vi "纳清叶绿素a电极校准.vi"() -> ()   [LabVIEW 2016, in "斯坦道多参数.lvlib"]
uses:
  <vilib>/Utility/miscctls.llb/LVPointTypeDef.ctl
  <vilib>/Utility/miscctls.llb/LVPositionTypeDef.ctl
  <vilib>/Analysis/NI_AALBase.lvlib
panel:
  out "滤波设定":sgl
  in  "量程":u16(ring) items=["0-500", "0-50"]
  out "第三点信号值":dbl
  out "第二点信号值":dbl
  out "第一点信号值":dbl
  out "报警信息":string
  out "通讯状态":string
  out "第三点校准值":dbl
  out "标液3":sgl
  out "第二点校准值":dbl
  out "第一点校准值":dbl
  in  "校准停止":bool
  in  "校准启动":bool
  in  "校准模式":u16(ring)=1 items=["两点校准", "单点校准", "三点校准"]
  out "最小值":sgl format="%#.2f"
  out "最大值":sgl format="%#.2f"
  out "波形图表":dbl(graph) caption="历史曲线"
  out "mean":dbl caption="均值" format="%#.2f"
  out "standard deviation":dbl caption="标准差" format="%#.2f"
  out "变异系数":dbl format="%#.6f"
  out "测量值":sgl format="%#.2f"
  out "提示":string
  out "标液2":sgl
  out "标液1":sgl
  out "原始光强数值":u16 caption="信号值"
  out "温度":dbl format="%#.2f"
  # "叶绿素a电极设定"
  # "℃"
  # "μg/L"
  # "μg/L"
  # "请选择校准模式:"
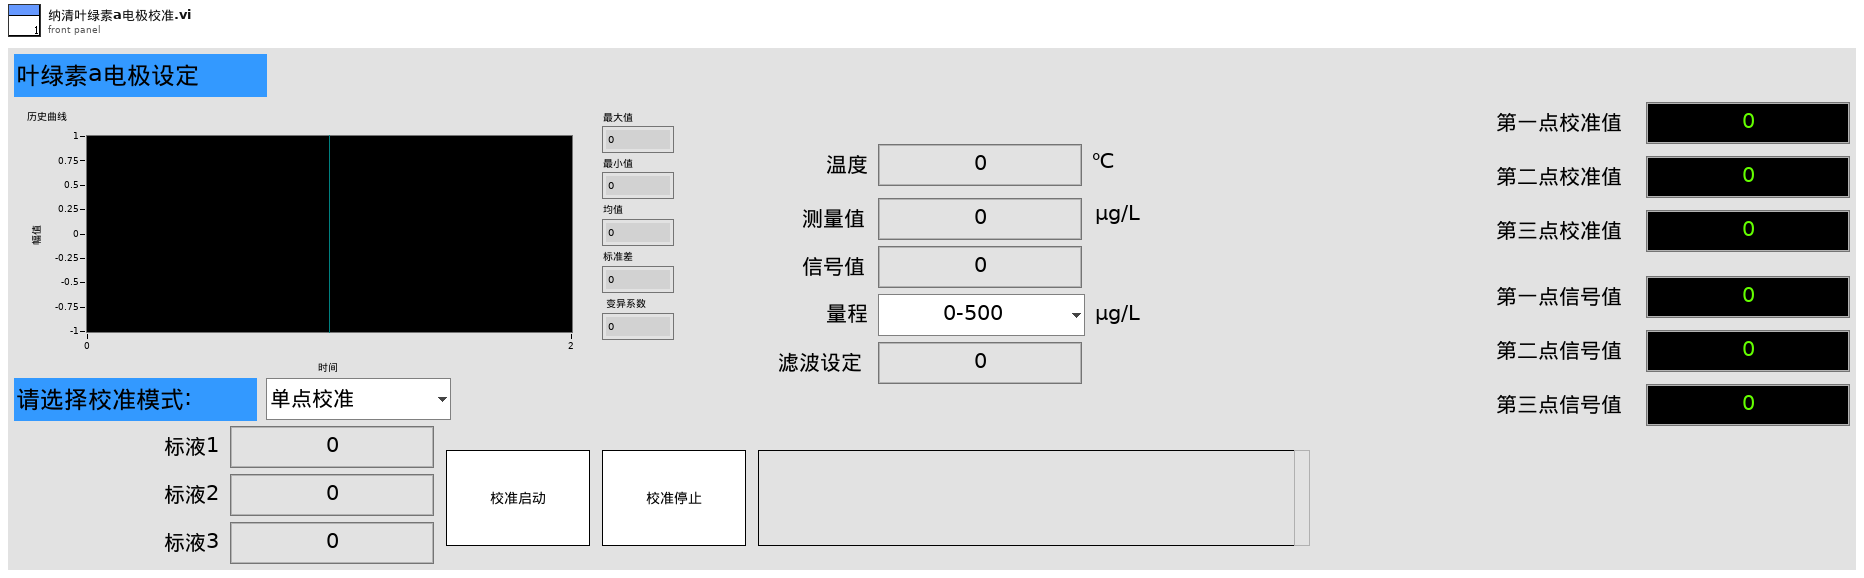
[diagram p1: front panel]
types:
  T1 = enum16{"pH", "DO", "Cond", "Turb", "ORP", "叶绿素a", "藻密度"}
  T2 = typedef "LVPointTypeDef.ctl" = cluster{"Horizontal":i16, "Vertical":i16}
  T3 = cluster{"报警码":u16, "叶绿素a":sgl, "温度数据":sgl, "原始光强数值":u16, "量程":u16, "平均次数":u16, "清扫模式":u16, "清扫次数":u16, "清扫间隔分钟":u16, "0X000B_NC":string, "产品名称":string, "序列号":string, "硬件版本":string, "软件版本":string, "通讯地址":u16, "波特率":u16, "设备类型":u16, "0X0026_NC":string, "校准量程":u16, "第一点原始光强":u16, "第一点校准数据":sgl, "第二点原始光强":u16, "第二点校准数据":sgl, "第三点原始光强":u16, "第三点校准数据":sgl, "探头校准命令":u16, "温度校准参数":sgl, "温度校准命令":u16}
  T4 = cluster{"pH":u32, "DO":u32, "Cond":u32, "Turb":u32, "叶绿素a":u32, "藻密度":u32, "ORP":u32}
  T5 = typedef "LVPositionTypeDef.ctl" = cluster{"Left":i32, "Top":i32}
  T6 = enum8{"Enabled", "Disabled", "Disabled and Grayed Out"}
  T7 = cluster{"ph":bool, "DO":bool, "Cond":bool, "Turb":bool, "叶绿素a":bool, "藻密度":bool, "ORP":bool}
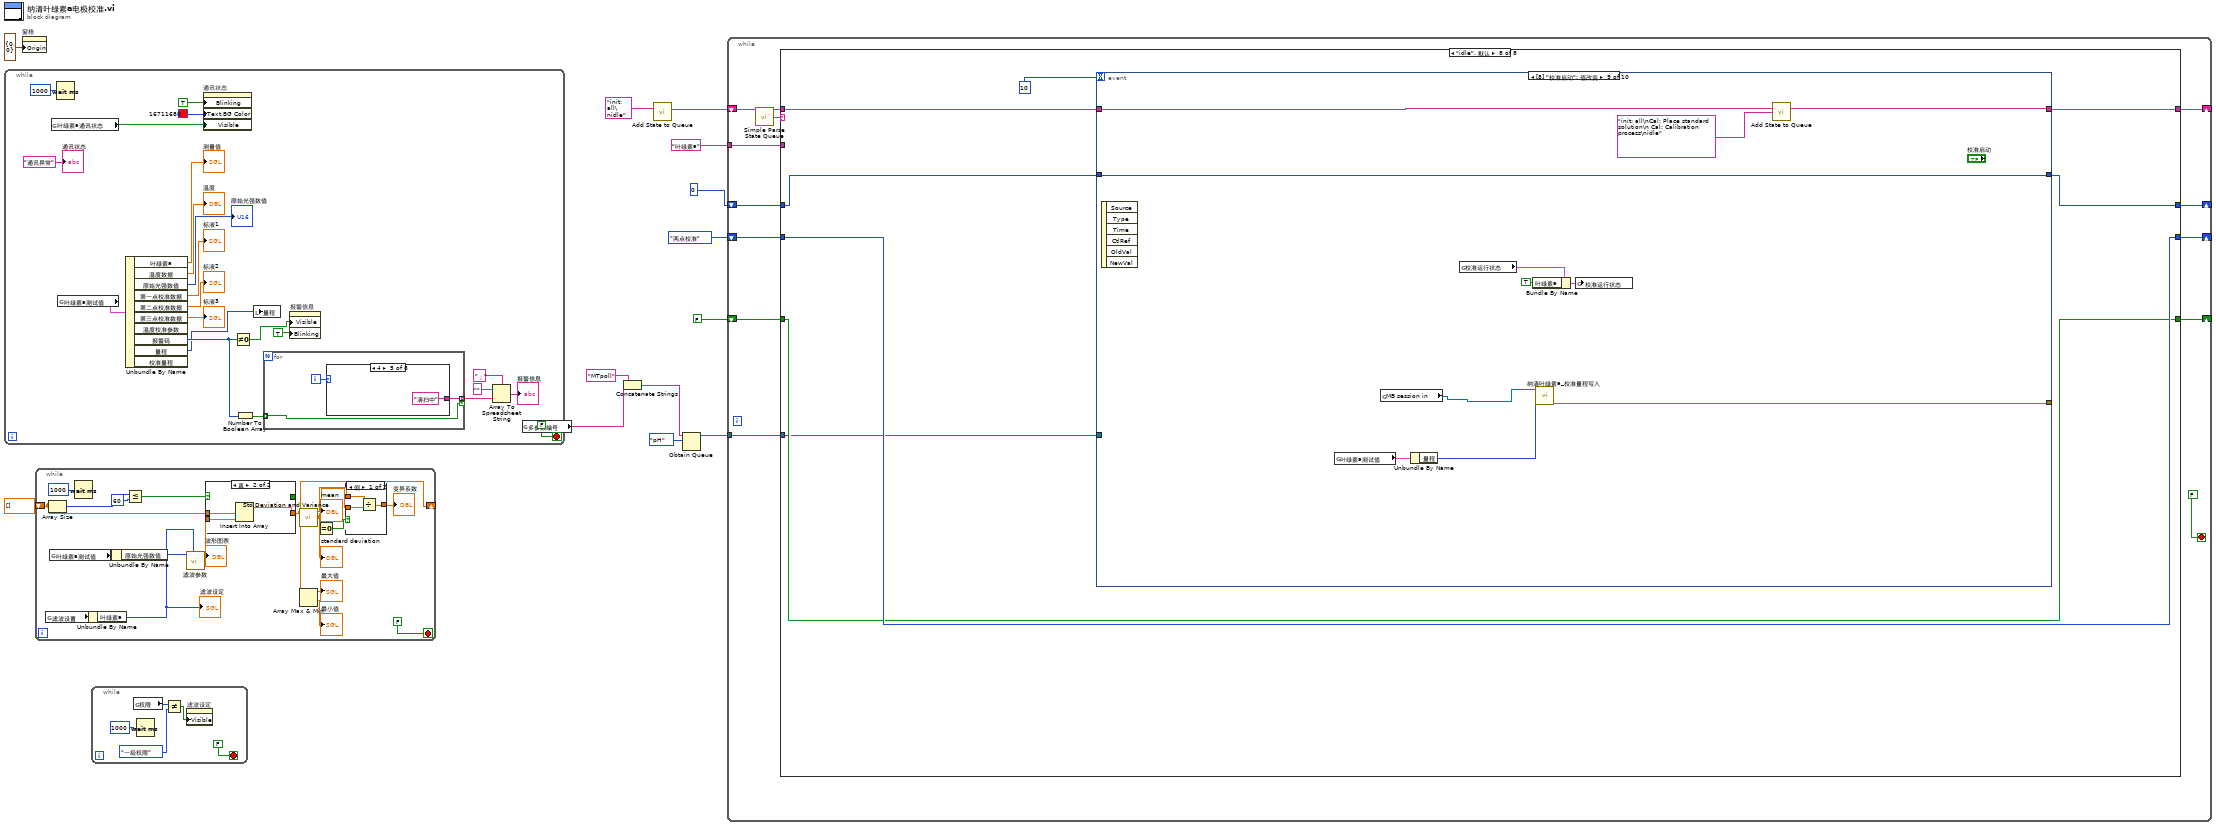
[diagram p0: block diagram]
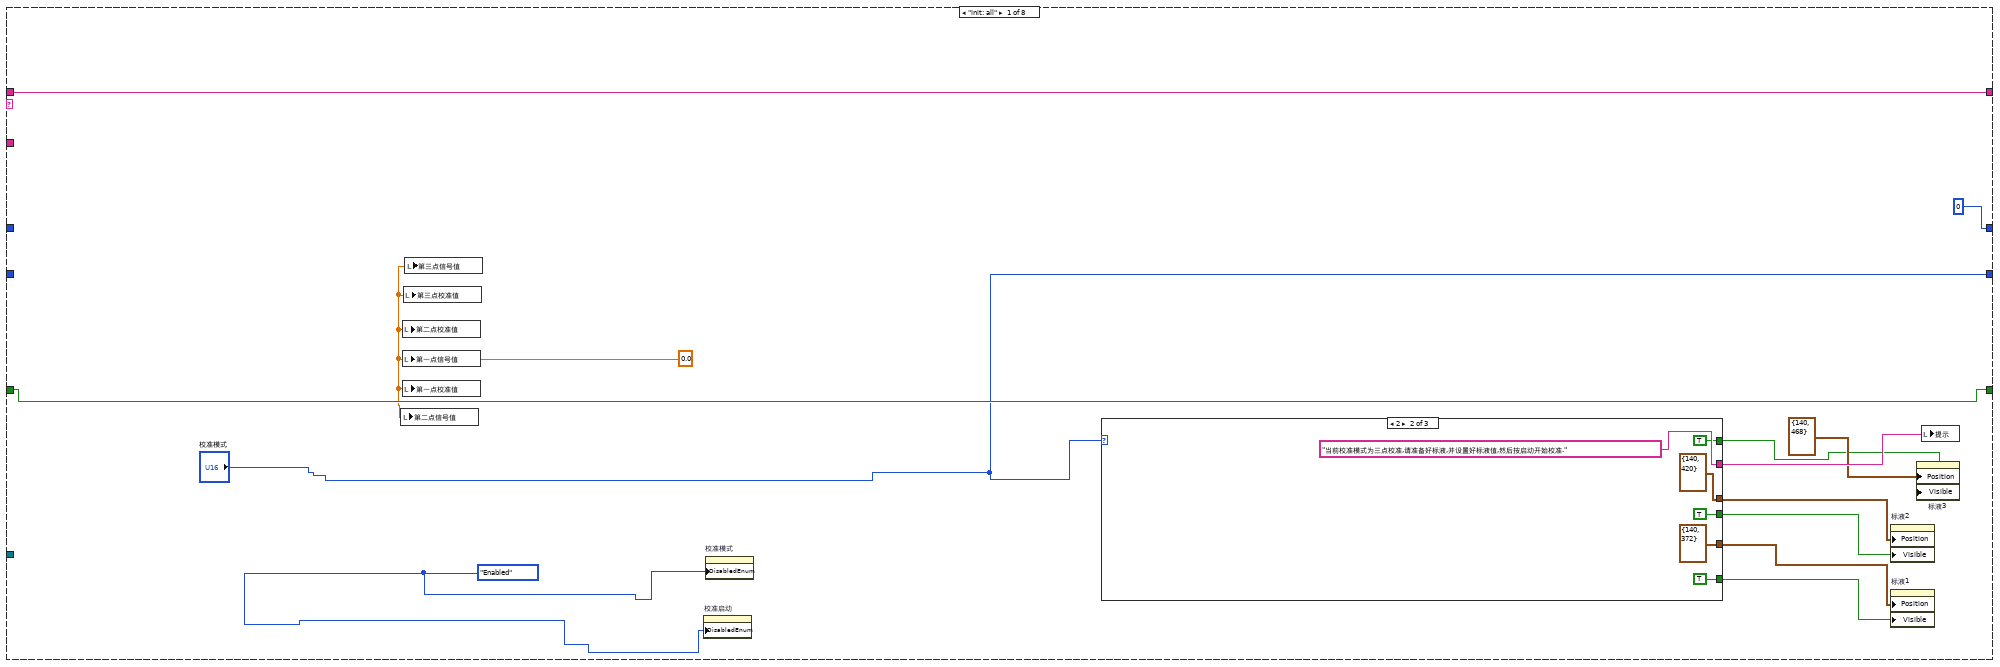
[diagram p2: hidden frame]
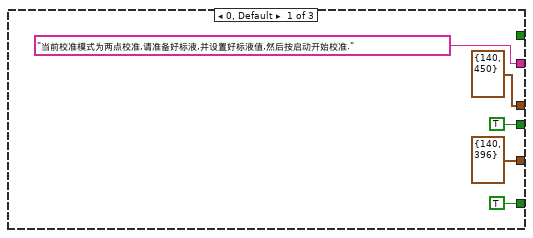
[diagram p3: hidden frame]
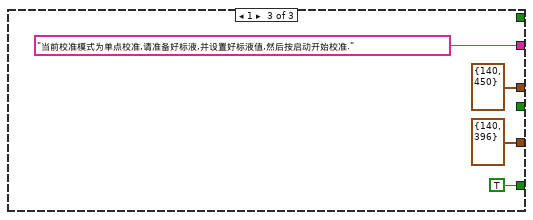
[diagram p4: hidden frame]
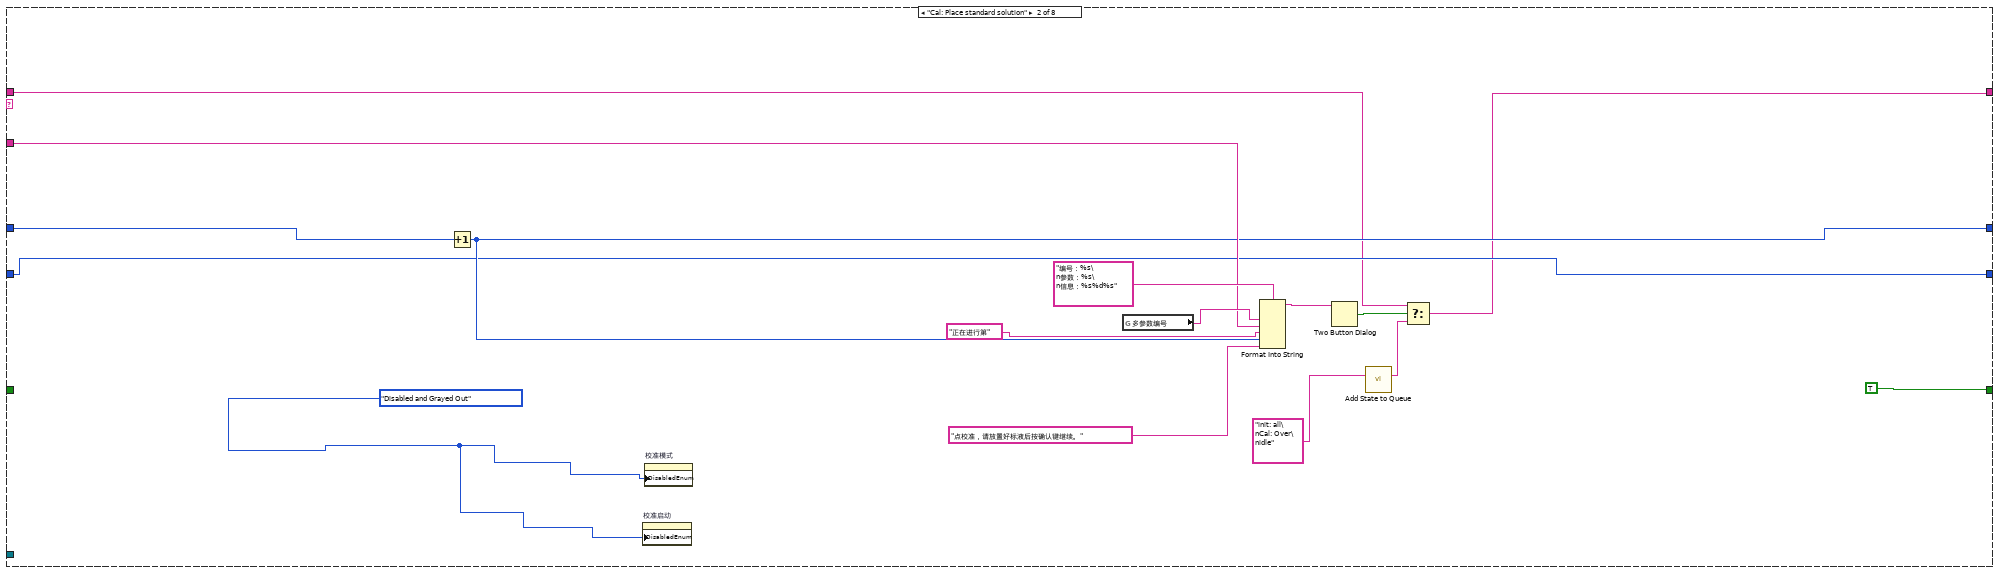
[diagram p5: hidden frame]
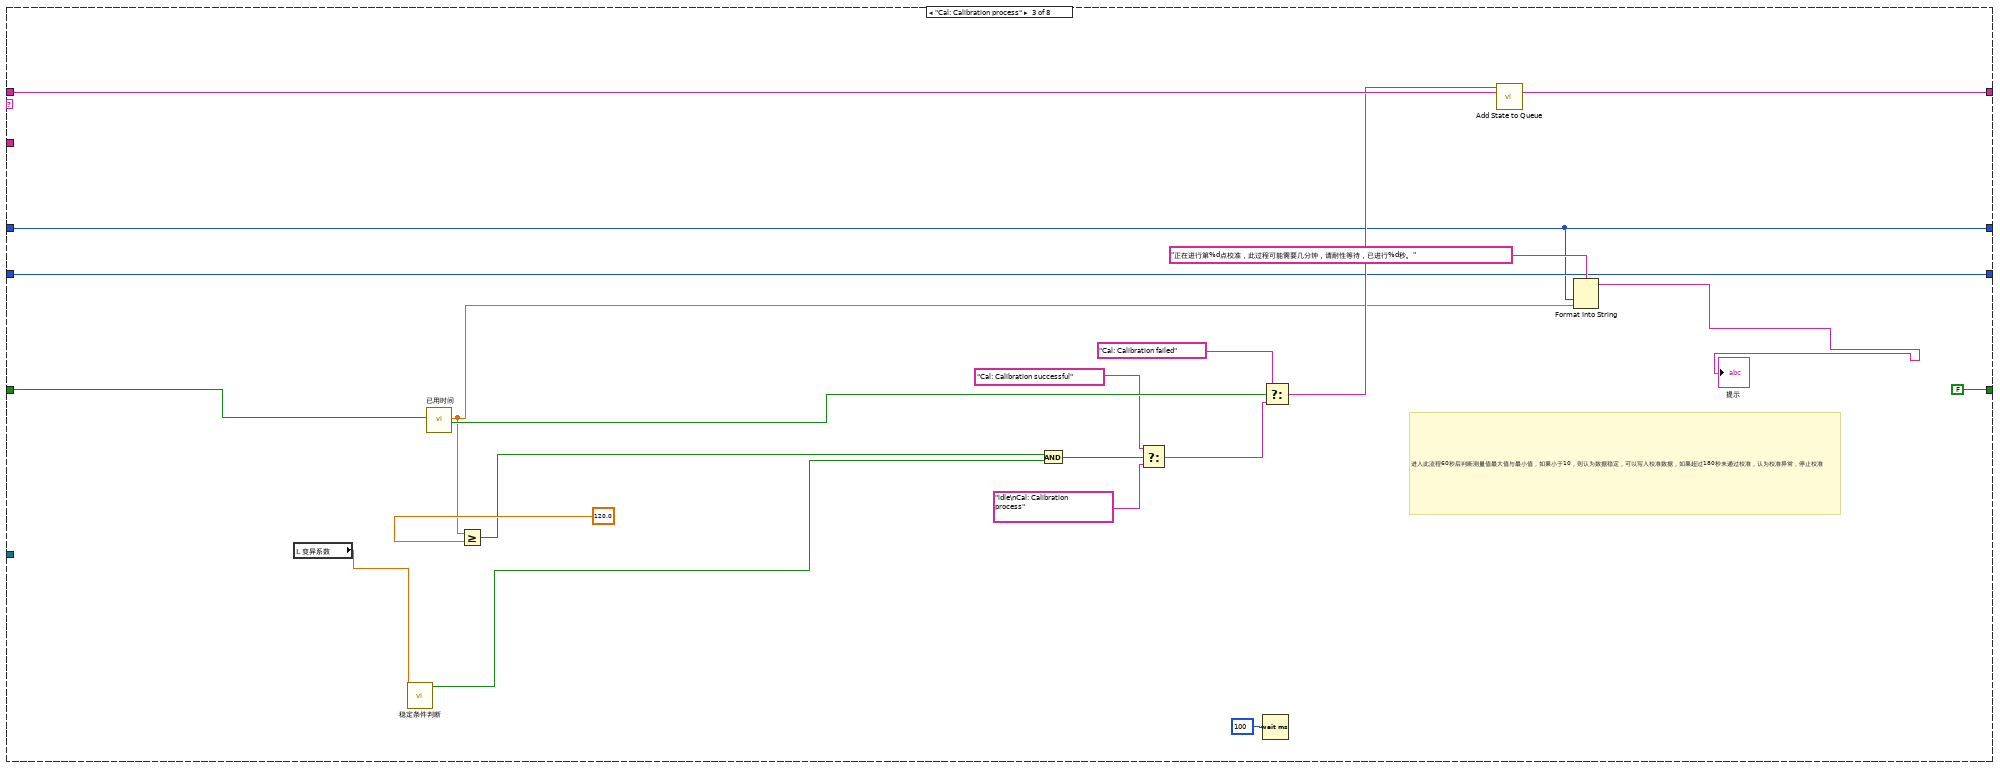
[diagram p6: hidden frame]
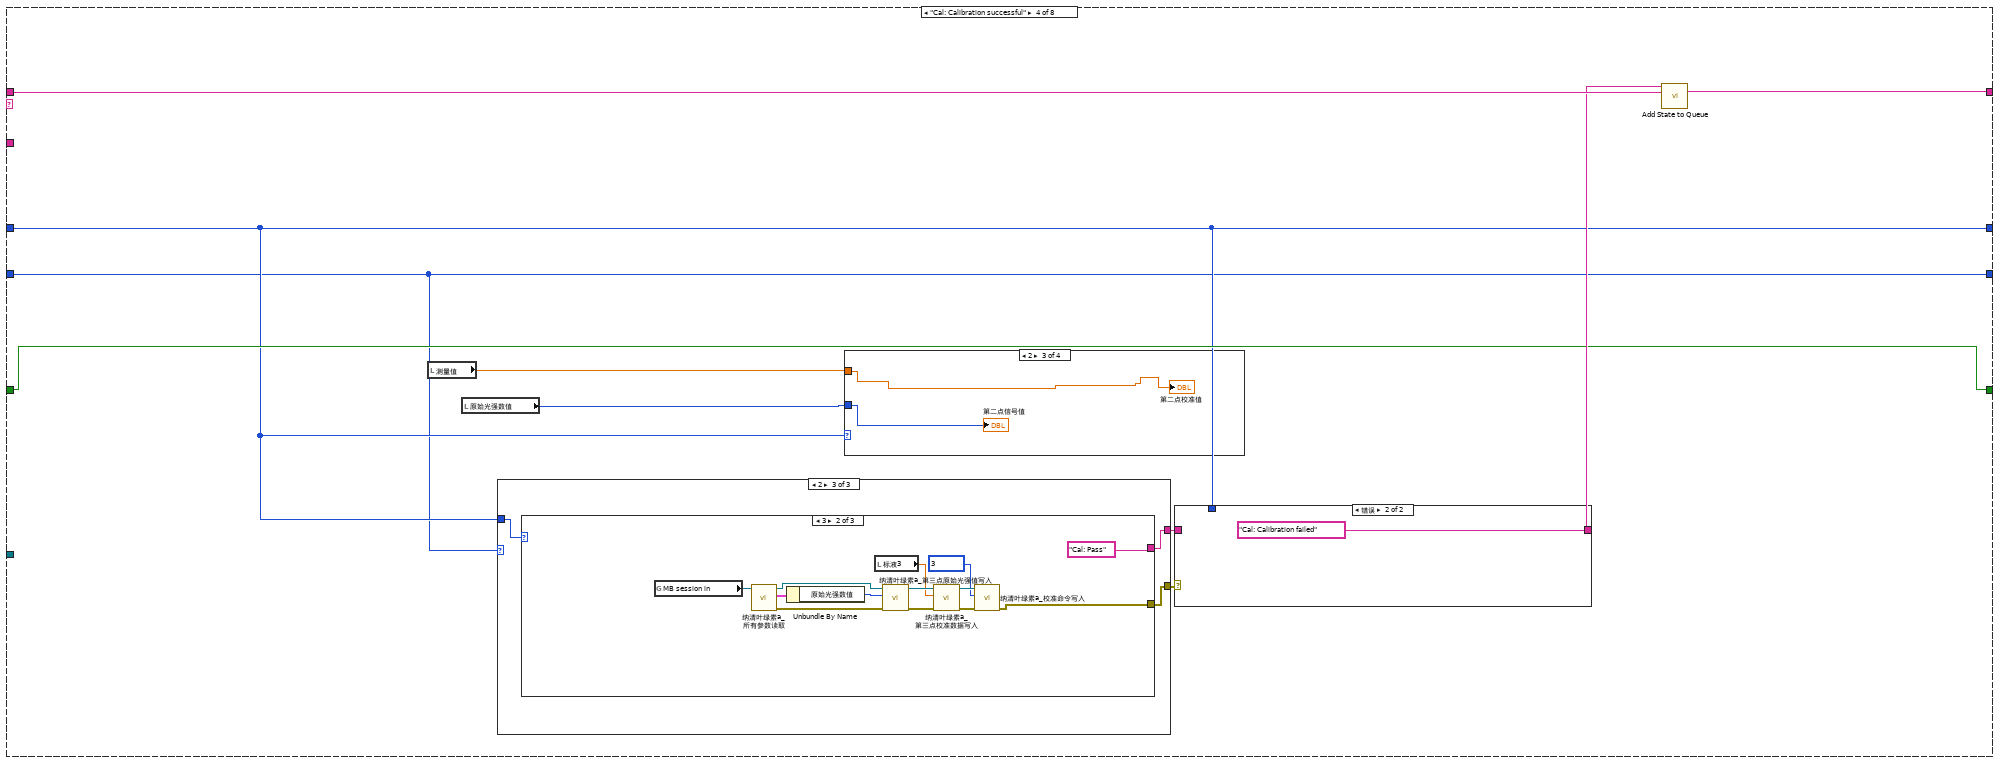
[diagram p7: hidden frame]
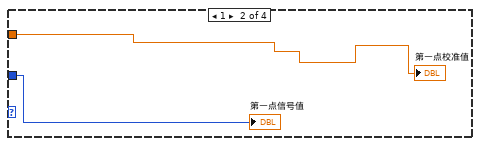
[diagram p9: hidden frame]
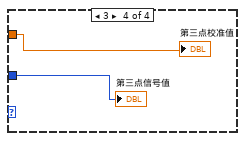
[diagram p10: hidden frame]
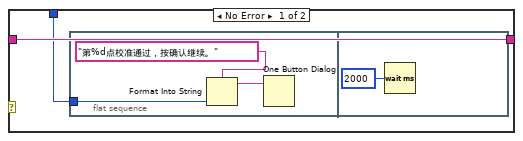
[diagram p11: hidden frame]
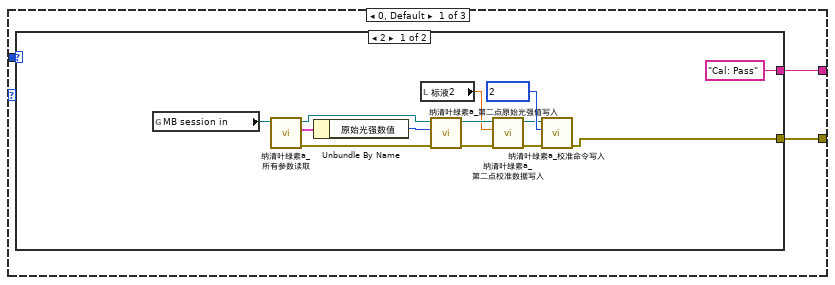
[diagram p12: hidden frame]
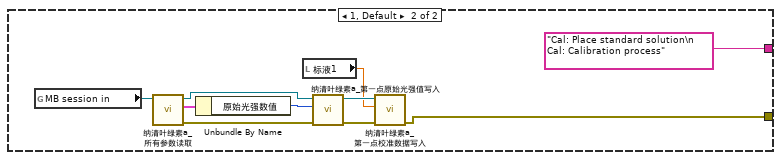
[diagram p13: hidden frame]
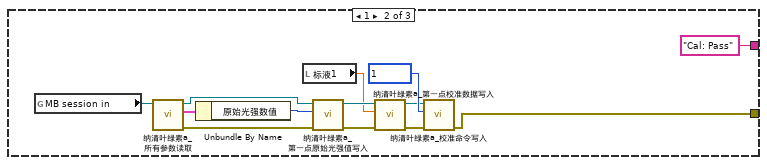
[diagram p14: hidden frame]
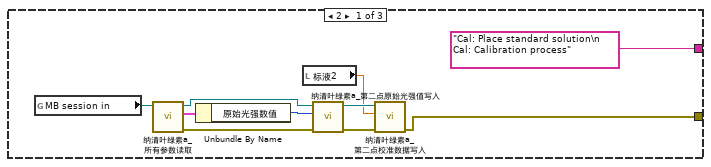
[diagram p15: hidden frame]
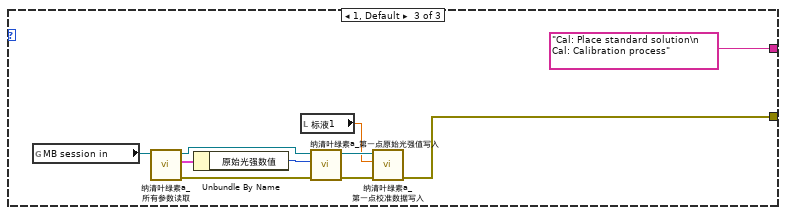
[diagram p16: hidden frame]
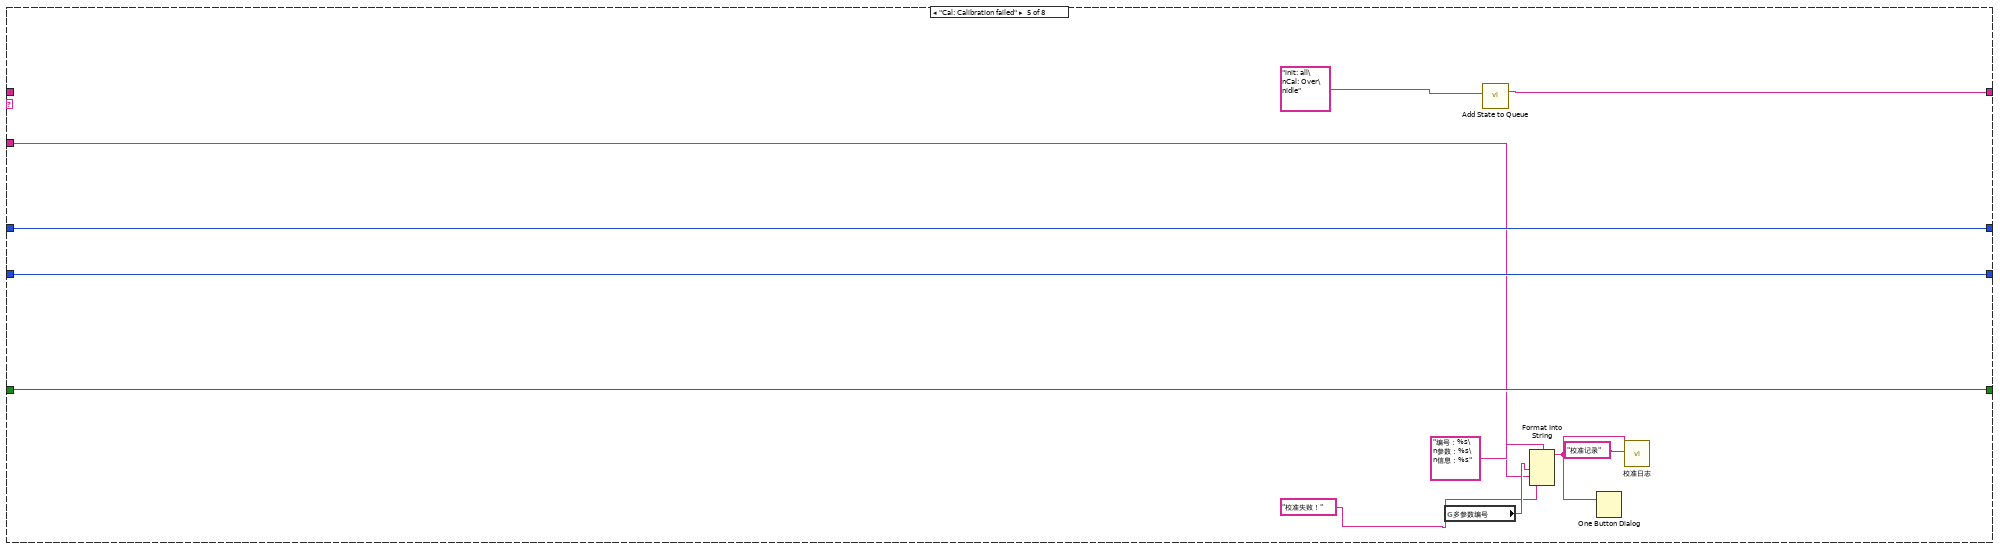
[diagram p17: hidden frame]
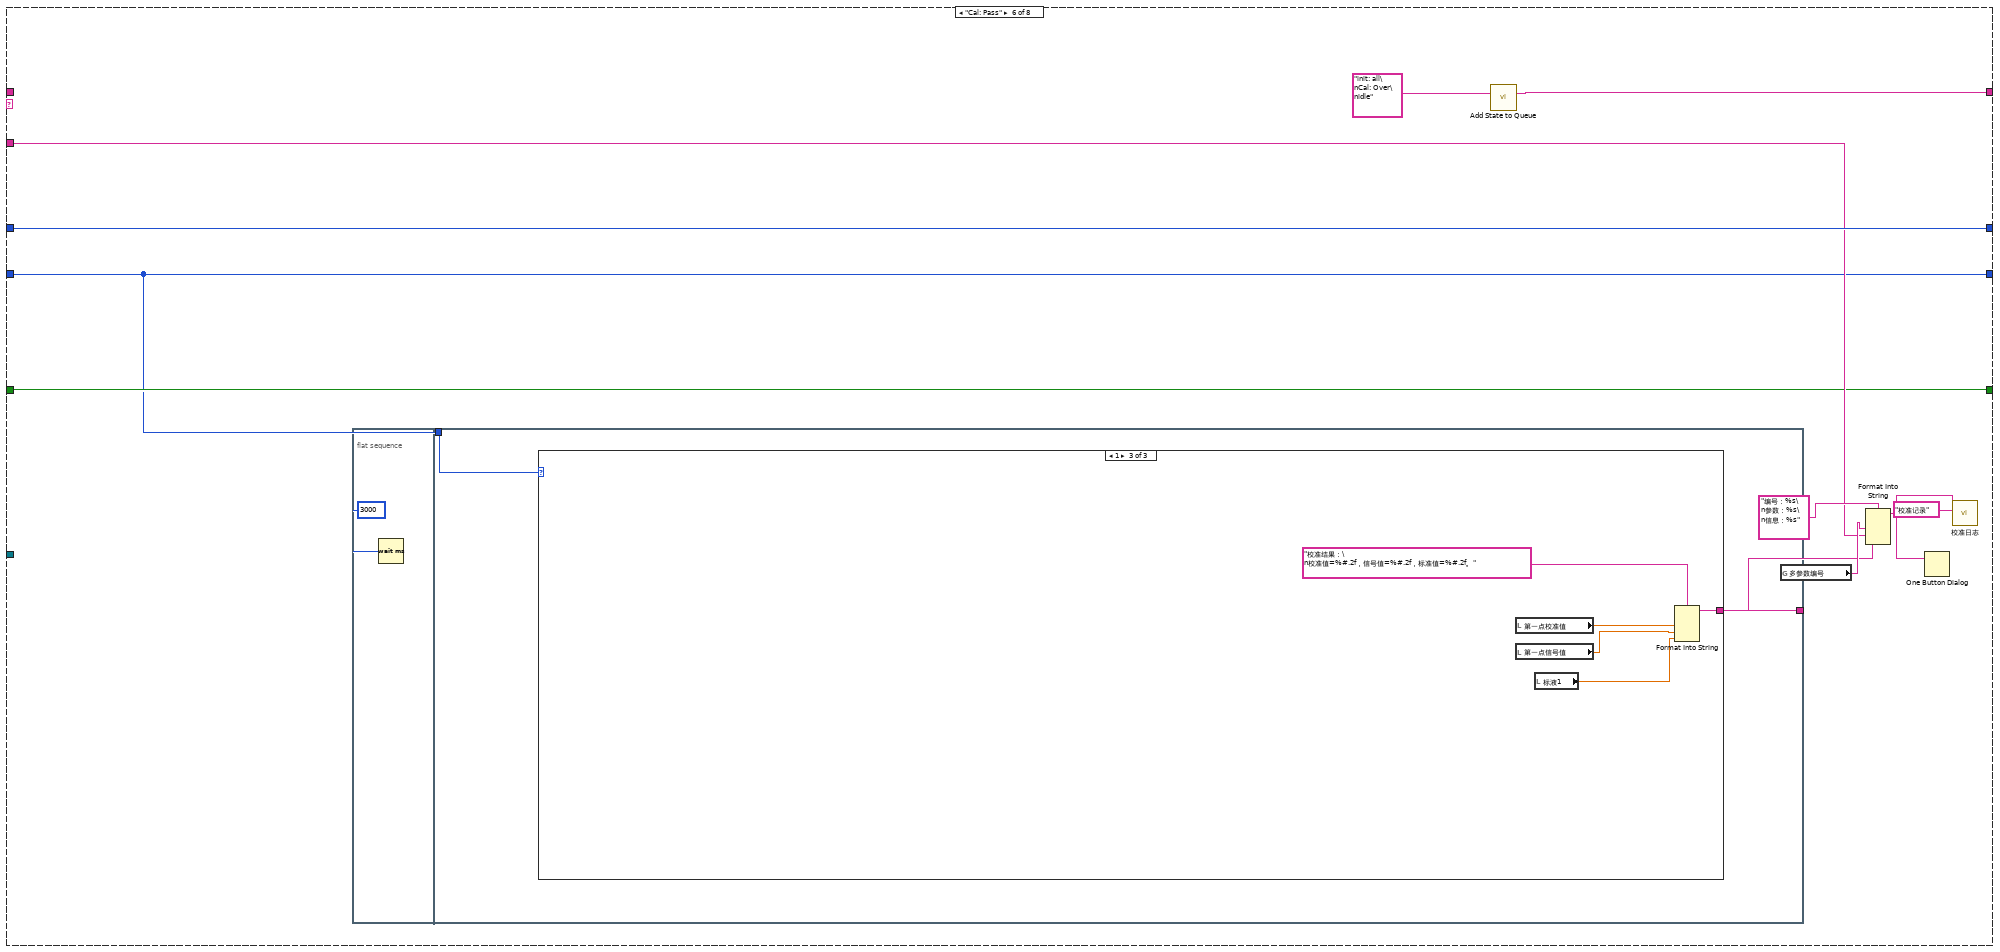
[diagram p18: hidden frame]
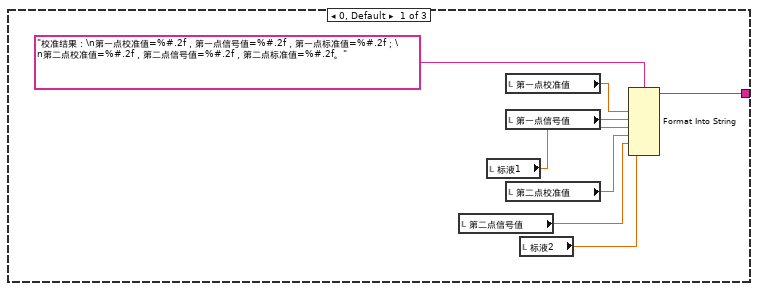
[diagram p19: hidden frame]
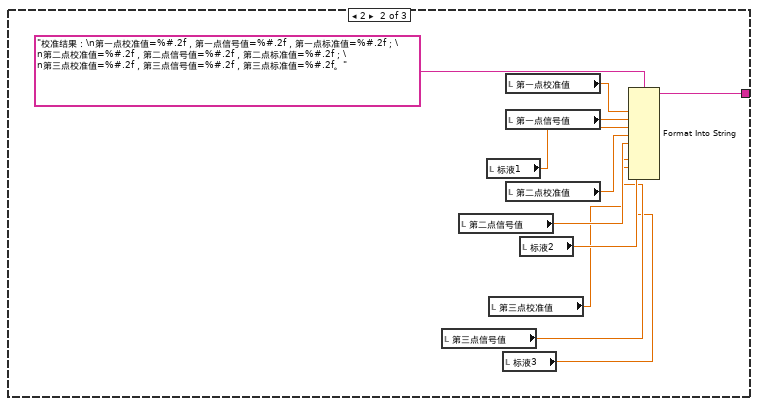
[diagram p20: hidden frame]
diagram:
  n1 = while {
    stop <- FALSE stop-if-true
    n2 = global read "多参数全局变量.vi" "叶绿素a通讯状态"() -> (w23:bool)
    n3 = Wait (ms)(milliseconds to wait=u32 1000 ("等待时间（毫秒）")) -> ()  [unwired: 1 out]
    n4 = global read "纳清过程全局变量.vi" "叶绿素a测试值"() -> (w33:T3)
    n5 = Unbundle By Name(w33) -> ("叶绿素a"=→"测量值":sgl, "温度数据"=→"温度":sgl, "原始光强数值"=→"原始光强数值":u16, "第一点校准数据"=→"标液1":sgl, "第二点校准数据"=→"标液2":sgl, "第三点校准数据"=→"标液3":sgl, "报警码"=w15:u16, "量程"=w14:u16)  [unwired: 2 out]
    n6 = property on="通讯状态" class="Str"("Blinking"=TRUE ("闪烁"), "Text.BG Color"=u32 16711680, "Visible"=w23) -> ()  [unwired: 2 in, 2 out]
    n7 = Not Equal To 0?(x=w15) -> (x != 0?=w17:bool)
    n8 = Number To Boolean Array(number=w15) -> (Boolean array=w22:bool[])
    n9 = local write "量程"(w14) -> ()
    n10 = for {
      tunnel: w22 -> [w36] mode=indexing
      tunnel: [w37] -> w21 mode=indexing if=w36
      i -> [w38]
      n11 = case shown="4" w38 {
        tunnel: [_ "浊度超量程" "温度超量程" "光强信号超范围" "清扫中" "温度传感器故障" "电极故障" "内部电压基准故障"] -> w37
        frame Default {
        }
        frame 0 {
        }
        frame 2 {
        }
        frame 3 {
        }
        frame 4 {
        }
        frame 8 {
        }
        frame 9 {
        }
        frame 10 {
        }
      }
    }
    n12 = property on="报警信息" class="Str"("Visible"=w17, "Blinking"=TRUE ("闪烁")) -> ()  [unwired: 2 in, 2 out]
    n13 = Array To Spreadsheet String(delimiter (Tab)="；" ("分隔符(Tab)"), array=w21, 3:"" ("格式字符串")) -> (spreadsheet string=→"报警信息":string)
    "通讯状态" <- "通讯异常" ("当前串口")
  }
  n14 = property on="窗格" class="Pane"("Origin"=T2 {"Horizontal"=0, "Vertical"=0} ("原点")) -> ()  [unwired: 2 in, 2 out]
  n15 = while {
    shift-right: [w53] -> _
    shift-left: sgl[] [] -> [w59]
    stop <- FALSE stop-if-true
    n16 = global read "断电保存变量.vi" "滤波设置"() -> (w47:T4)
    n17 = Array Size(array=w59) -> (size(s)=w61:i32)
    n18 = global read "纳清过程全局变量.vi" "叶绿素a测试值"() -> (w50:T3)
    n19 = Wait (ms)(milliseconds to wait=u32 1000 ("等待时间（毫秒）")) -> ()  [unwired: 1 out]
    n20 = Unbundle By Name(w47) -> ("叶绿素a"=w46:u32)
    "滤波设定" <- w46
    n21 = Unbundle By Name(w50) -> ("原始光强数值"=w49:u16)
    n22 = Less Or Equal?(x=w61, y=60) -> (x <= y?=w60:bool)
    n23 = call "滤波参数.vi"("滤波次数"=w46, "x"=w49) -> ("mode"=w48:dbl)  [unwired: 9 in]
    "波形图表" <- w48
    n24 = case shown="真" w60 {
      tunnel: w59 -> [w72 w75]
      tunnel: w48 -> [w70 w74]
      tunnel: [w68 w73] -> w53
      tunnel: [TRUE _] -> _
      frame False {
        n25 = Replace Array Subset(array=w72, new element=w70) -> (w71:sgl[])  [unwired: 1 in]
        n26 = Rotate 1D Array(1:w71, 2:-1 ("n")) -> (0:w68:sgl[])
      }
      frame True {
        n27 = Insert Into Array(array=w75, new element=w74) -> (w73:sgl[])  [unwired: 1 in]
      }
    }
    n28 = call <vilib>:"Std Deviation and Variance.vi"("X"=w53) -> ("mean"=w57:dbl, "standard deviation"=w56:dbl)  [unwired: 1 in, 1 out]
    "mean" <- w57
    "standard deviation" <- w56
    n29 = Array Max & Min(array=w53) -> (max value=→"最大值":sgl, min value=→"最小值":sgl)  [unwired: 2 out]
    n30 = Equal To 0?(x=w57) -> (x = 0?=w58:bool)
    n31 = case shown="假" w58 {
      tunnel: w56 -> [w66 _]
      tunnel: [w65 _] -> w55
      tunnel: w57 -> [w64 _]
      frame False {
        n32 = Divide(x=w66, y=w64) -> (x/y=w65:dbl)
      }
      frame True {
      }
    }
    "变异系数" <- w55
  }
  n33 = while {
    stop <- FALSE stop-if-true
    n34 = global read "多参数全局变量.vi" "权限"() -> (w79:enum16{"一级权限", "二级权限", "三级权限"})
    n35 = Wait (ms)(milliseconds to wait=u32 1000 ("等待时间（毫秒）")) -> ()  [unwired: 1 out]
    n36 = Not Equal?(x=w79, y=enum16{"一级权限", "二级权限", "三级权限"}."一级权限") -> (x != y?=w76:bool)
    n37 = property on="滤波设定" class="DigNum (严格)"("Visible"=w76) -> ()  [unwired: 2 in, 2 out]
  }
  n38 = global read "多参数全局变量.vi" "多参数编号"() -> (w2:string)
  n39 = Concatenate Strings("MTpoll" ("名称（未命名）"), w2) -> (w4:string)
  n40 = call "Add State to Queue.vi"("State(s) In (\"\")"="init: all\nidle" ("State(s) In (\"\")")) -> ("States Out"=w10:string)  [unwired: 14 in]
  n41 = Obtain Queue(name (unnamed)=w4, element data type=T1."pH" ("枚举")) -> (queue out=w1:refnum<queue>)  [unwired: 3 in, 2 out]
  n42 = while {
    shift-right: [w89] -> _
    shift-left: w10 -> [w93]
    shift-right: [w86] -> _
    shift-left: 0 -> [w88]
    tunnel: "叶绿素a" ("State(s) In (\"\")") -> [w87]
    shift-right: [w84] -> _
    shift-left: enum16{"两点校准", "单点校准", "三点校准"}."两点校准" ("校准模式") -> [w85]
    shift-right: [w82] -> _
    shift-left: FALSE -> [w83]
    tunnel: w1 -> [w81]
    stop <- FALSE stop-if-true
    n43 = call "Simple Parse State Queue.vi"("State Queue"=w93) -> ("Remain States"=w90:string, "Next State"=w91:string)  [unwired: 13 in]
    n44 = case shown="\"idle\", 默认" w91 {
      tunnel: w90 -> [w106 w125 w157 w166 _ _ w312 w320]
      tunnel: [w106 w124 w156 w165 w264 w269 w312 w319] -> w89
      tunnel: w88 -> [_ w133 w142 w160 w267 w278 w311 w317]
      tunnel: w87 -> [_ w134 _ _ w258 w274 _ _]
      tunnel: [0 w131 w142 w160 w267 w278 w311 w318] -> w86
      tunnel: w85 -> [_ w130 w143 w159 w266 w270 w310 w316]
      tunnel: ["校准模式" w130 w143 w159 w266 w270 w310 w316] -> w84
      tunnel: w83 -> [w104 _ w145 w161 w265 w273 w309 w314]
      tunnel: [w104 TRUE FALSE w161 w265 w273 w309 w314] -> w82
      tunnel: w81 -> [_ _ _ _ _ _ _ w313]
      frame "init: all" {
        w101 = T6."Enabled" ("禁用")
        w103 = 0.0 ("第一点校准值")
        n45 = local write "第二点信号值"(w103) -> ()
        n46 = local write "第二点校准值"(w103) -> ()
        n47 = local write "第一点信号值"(w103) -> ()
        n48 = local write "第一点校准值"(w103) -> ()
        n49 = local write "第三点校准值"(w103) -> ()
        n50 = local write "第三点信号值"(w103) -> ()
        n51 = property on="校准启动" class="Bool"("DisabledEnum"=w101) -> ()  [unwired: 2 in, 2 out]
        n52 = property on="校准模式" class="Ring (严格)"("DisabledEnum"=w101) -> ()  [unwired: 2 in, 2 out]
        n53 = case shown="2" "校准模式" {
          tunnel: ["当前校准模式为两点校准,请准备好标液,并设置好标液值,然后按启动开始校准." ("提示") "当前校准模式为三点校准,请准备好标液,并设置好标液值,然后按启动开始校准." ("提示") "当前校准模式为单点校准,请准备好标液,并设置好标液值,然后按启动开始校准." ("提示")] -> w102
          tunnel: [TRUE ("可见") TRUE ("可见") _] -> w96
          tunnel: [T5 {"Left"=140, "Top"=396} ("位置") T5 {"Left"=140, "Top"=372} ("位置") T5 {"Left"=140, "Top"=396} ("位置")] -> w95
          tunnel: [T5 {"Left"=140, "Top"=450} ("位置 2") T5 {"Left"=140, "Top"=420} ("位置 2") T5 {"Left"=140, "Top"=450} ("位置 2")] -> w97
          tunnel: [_ TRUE ("可见") _] -> w98
          tunnel: [TRUE ("可见") TRUE ("可见") TRUE ("可见")] -> w94
          frame 0, Default {
          }
          frame 2 {
          }
          frame 1 {
          }
        }
        n54 = property on="标液2" class="DigNum (严格)"("Position"=w97, "Visible"=w96) -> ()  [unwired: 2 in, 2 out]
        n55 = property on="标液1" class="DigNum (严格)"("Position"=w95, "Visible"=w94) -> ()  [unwired: 2 in, 2 out]
        n56 = property on="标液3" class="DigNum (严格)"("Position"=T5 {"Left"=140, "Top"=468} ("位置 3"), "Visible"=w98) -> ()  [unwired: 2 in, 2 out]
        n57 = local write "提示"(w102) -> ()
      }
      frame "Cal: Place standard solution" {
        w123 = T6."Disabled and Grayed Out" ("禁用")
        n58 = Increment(x=w133) -> (x+1=w131:i32)
        n59 = property on="校准启动" class="Bool"("DisabledEnum"=w123) -> ()  [unwired: 2 in, 2 out]
        n60 = property on="校准模式" class="Ring (严格)"("DisabledEnum"=w123) -> ()  [unwired: 2 in, 2 out]
        n61 = global read "多参数全局变量.vi" "多参数编号"() -> (w136:string)
        n62 = Format Into String(format string="编号：%s\n参数：%s\n信息：%s%d%s" ("格式字符串"), w136, w134, "正在进行第" ("消息"), w131, "点校准，请放置好标液后按确认键继续。" ("消息")) -> (resulting string=w128:string)  [unwired: 2 in, 1 out]
        n63 = Two Button Dialog(message=w128) -> (T button?=w127:bool)  [unwired: 2 in]
        n64 = call "Add State to Queue.vi"("State(s) In (\"\")"="init: all\nCal: Over\nidle" ("State(s) In (\"\")")) -> ("States Out"=w126:string)  [unwired: 14 in]
        n65 = Select(t=w125, s=w127, f=w126) -> (s? t:f=w124:string)
      }
      frame "Cal: Calibration process" {
        # "进入此流程60秒后判断测量值最大值与最小值，如果小于10，则认为数据稳定，可以写入校准数据，如果超过180秒未通过校准，认为校准异常，停止校准"
        n66 = local read "变异系数"() -> (w139:dbl)
        n67 = call "稳定条件判断.vi"("变异系数"=w139) -> ("布尔"=w138:bool)  [unwired: 10 in]
        n68 = call "已用时间"("Reset"=w145) -> ("Elapsed Time (s)"=w141:dbl, "Time has Elapsed"=w158:bool)  [unwired: 11 in, 6 out]
        n69 = Greater Or Equal?(x=w141, y=120.0) -> (x >= y?=w153:bool)
        n70 = And(x=w153, y=w138) -> (x .and. y?=w150:bool)
        n71 = Select(t="Cal: Calibration successful" ("State(s) In (\"\")"), s=w150, f="idle\nCal: Calibration process" ("State(s) In (\"\")")) -> (s? t:f=w149:string)
        n72 = Wait (ms)(milliseconds to wait=u32 100 ("等待时间（毫秒）")) -> ()  [unwired: 1 out]
        n73 = Select(t="Cal: Calibration failed" ("State(s) In (\"\")"), s=w158, f=w149) -> (s? t:f=w148:string)
        n74 = call "Add State to Queue.vi"("State(s) In Front (\"\")"=w148, "State(s) In (\"\")"=w157) -> ("States Out"=w156:string)  [unwired: 13 in]
        n75 = Format Into String(format string="正在进行第%d点校准，此过程可能需要几分钟，请耐性等待，已进行%d秒。" ("格式字符串"), w142, w141) -> (resulting string=→"提示":string)  [unwired: 2 in, 1 out]
      }
      frame "Cal: Calibration successful" {
        n76 = local read "测量值"() -> (w162:sgl)
        n77 = local read "原始光强数值"() -> (w163:u16)
        n78 = case shown="2" w159 {
          tunnel: [w184 w208 w221] -> w168
          tunnel: [w183 "Cal: Pass" ("State(s) In (\"\")") w222] -> w167
          tunnel: w160 -> [w182 _ w223]
          frame 0, Default {
            n79 = case shown="2" w182 {
              tunnel: [w185 w198] -> w184
              tunnel: ["Cal: Pass" ("State(s) In (\"\")") "Cal: Place standard solution\n Cal: Calibration process" ("State(s) In (\"\")")] -> w183
              frame 2 {
                n80 = global read "多参数全局变量.vi" "MB session in"() -> (w193:refnum<class "MB_Master.lvclass">)
                n81 = call "纳清叶绿素a_所有参数读取.vi"("MB session in"=w193) -> ("error out"=w195:errorcluster, "输出值"=w192:T3, "MB session out"=w194:refnum<class "MB_Master.lvclass">)  [unwired: 8 in]
                n82 = Unbundle By Name(w192) -> ("原始光强数值"=w191:u16)
                n83 = local read "标液2"() -> (w186:sgl)
                n84 = call "纳清叶绿素a_第二点原始光强值写入.vi"("error in (no error)"=w195, "数值"=w191, "MB session in"=w194) -> ("error out"=w190:errorcluster, "MB session out"=w189:refnum<class "MB_Master.lvclass">)  [unwired: 7 in]
                n85 = call "纳清叶绿素a_第二点校准数据写入.vi"("error in (no error)"=w190, "数值"=w186, "MB session in"=w189) -> ("error out"=w188:errorcluster, "MB session out"=w187:refnum<class "MB_Master.lvclass">)  [unwired: 7 in]
                n86 = call "纳清叶绿素a_校准命令写入.vi"("error in (no error)"=w188, "数值"=u16 2 ("starting address"), "MB session in"=w187) -> ("error out"=w185:errorcluster)  [unwired: 7 in, 1 out]
              }
              frame 1, Default {
                n87 = global read "多参数全局变量.vi" "MB session in"() -> (w204:refnum<class "MB_Master.lvclass">)
                n88 = call "纳清叶绿素a_所有参数读取.vi"("MB session in"=w204) -> ("error out"=w206:errorcluster, "输出值"=w203:T3, "MB session out"=w205:refnum<class "MB_Master.lvclass">)  [unwired: 8 in]
                n89 = Unbundle By Name(w203) -> ("原始光强数值"=w202:u16)
                n90 = local read "标液1"() -> (w199:sgl)
                n91 = call "纳清叶绿素a_第一点原始光强值写入.vi"("error in (no error)"=w206, "数值"=w202, "MB session in"=w205) -> ("error out"=w201:errorcluster, "MB session out"=w200:refnum<class "MB_Master.lvclass">)  [unwired: 7 in]
                n92 = call "纳清叶绿素a_第一点校准数据写入.vi"("error in (no error)"=w201, "数值"=w199, "MB session in"=w200) -> ("error out"=w198:errorcluster)  [unwired: 7 in, 1 out]
              }
            }
          }
          frame 1 {
            n93 = global read "多参数全局变量.vi" "MB session in"() -> (w216:refnum<class "MB_Master.lvclass">)
            n94 = call "纳清叶绿素a_所有参数读取.vi"("MB session in"=w216) -> ("error out"=w218:errorcluster, "输出值"=w215:T3, "MB session out"=w217:refnum<class "MB_Master.lvclass">)  [unwired: 8 in]
            n95 = Unbundle By Name(w215) -> ("原始光强数值"=w214:u16)
            n96 = local read "标液1"() -> (w209:sgl)
            n97 = call "纳清叶绿素a_第一点原始光强值写入.vi"("error in (no error)"=w218, "数值"=w214, "MB session in"=w217) -> ("error out"=w213:errorcluster, "MB session out"=w212:refnum<class "MB_Master.lvclass">)  [unwired: 7 in]
            n98 = call "纳清叶绿素a_第一点校准数据写入.vi"("error in (no error)"=w213, "数值"=w209, "MB session in"=w212) -> ("error out"=w211:errorcluster, "MB session out"=w210:refnum<class "MB_Master.lvclass">)  [unwired: 7 in]
            n99 = call "纳清叶绿素a_校准命令写入.vi"("error in (no error)"=w211, "数值"=u16 1 ("starting address"), "MB session in"=w210) -> ("error out"=w208:errorcluster)  [unwired: 7 in, 1 out]
          }
          frame 2 {
            n100 = case shown="3" w223 {
              tunnel: [w224 w234 w247] -> w221
              tunnel: ["Cal: Place standard solution\n Cal: Calibration process" ("State(s) In (\"\")") "Cal: Pass" ("State(s) In (\"\")") "Cal: Place standard solution\n Cal: Calibration process" ("State(s) In (\"\")")] -> w222
              frame 2 {
                n101 = global read "多参数全局变量.vi" "MB session in"() -> (w230:refnum<class "MB_Master.lvclass">)
                n102 = call "纳清叶绿素a_所有参数读取.vi"("MB session in"=w230) -> ("error out"=w232:errorcluster, "输出值"=w229:T3, "MB session out"=w231:refnum<class "MB_Master.lvclass">)  [unwired: 8 in]
                n103 = Unbundle By Name(w229) -> ("原始光强数值"=w228:u16)
                n104 = local read "标液2"() -> (w225:sgl)
                n105 = call "纳清叶绿素a_第二点原始光强值写入.vi"("error in (no error)"=w232, "数值"=w228, "MB session in"=w231) -> ("error out"=w227:errorcluster, "MB session out"=w226:refnum<class "MB_Master.lvclass">)  [unwired: 7 in]
                n106 = call "纳清叶绿素a_第二点校准数据写入.vi"("error in (no error)"=w227, "数值"=w225, "MB session in"=w226) -> ("error out"=w224:errorcluster)  [unwired: 7 in, 1 out]
              }
              frame 3 {
                n107 = global read "多参数全局变量.vi" "MB session in"() -> (w243:refnum<class "MB_Master.lvclass">)
                n108 = call "纳清叶绿素a_所有参数读取.vi"("MB session in"=w243) -> ("error out"=w245:errorcluster, "输出值"=w242:T3, "MB session out"=w244:refnum<class "MB_Master.lvclass">)  [unwired: 8 in]
                n109 = Unbundle By Name(w242) -> ("原始光强数值"=w241:u16)
                n110 = local read "标液3"() -> (w235:sgl)
                n111 = call "纳清叶绿素a_第三点原始光强值写入.vi"("error in (no error)"=w245, "数值"=w241, "MB session in"=w244) -> ("error out"=w240:errorcluster, "MB session out"=w239:refnum<class "MB_Master.lvclass">)  [unwired: 7 in]
                n112 = call "纳清叶绿素a_第三点校准数据写入.vi"("error in (no error)"=w240, "数值"=w235, "MB session in"=w239) -> ("error out"=w238:errorcluster, "MB session out"=w237:refnum<class "MB_Master.lvclass">)  [unwired: 7 in]
                n113 = call "纳清叶绿素a_校准命令写入.vi"("error in (no error)"=w238, "数值"=u16 3 ("starting address"), "MB session in"=w237) -> ("error out"=w234:errorcluster)  [unwired: 7 in, 1 out]
              }
              frame 1, Default {
                n114 = global read "多参数全局变量.vi" "MB session in"() -> (w253:refnum<class "MB_Master.lvclass">)
                n115 = call "纳清叶绿素a_所有参数读取.vi"("MB session in"=w253) -> ("error out"=w255:errorcluster, "输出值"=w252:T3, "MB session out"=w254:refnum<class "MB_Master.lvclass">)  [unwired: 8 in]
                n116 = Unbundle By Name(w252) -> ("原始光强数值"=w251:u16)
                n117 = local read "标液1"() -> (w248:sgl)
                n118 = call "纳清叶绿素a_第一点原始光强值写入.vi"("error in (no error)"=w255, "数值"=w251, "MB session in"=w254) -> ("error out"=w250:errorcluster, "MB session out"=w249:refnum<class "MB_Master.lvclass">)  [unwired: 7 in]
                n119 = call "纳清叶绿素a_第一点校准数据写入.vi"("error in (no error)"=w250, "数值"=w248, "MB session in"=w249) -> ("error out"=w247:errorcluster)  [unwired: 7 in, 1 out]
              }
            }
          }
        }
        n120 = case shown="2" w160 {
          tunnel: w163 -> [_ w170 w172 w174]
          tunnel: w162 -> [_ w169 w171 w173]
          frame 0, Default {
          }
          frame 1 {
            "第一点信号值" <- w170
            "第一点校准值" <- w169
          }
          frame 2 {
            "第二点信号值" <- w172
            "第二点校准值" <- w171
          }
          frame 3 {
            "第三点信号值" <- w174
            "第三点校准值" <- w173
          }
        }
        n121 = case shown="错误" w168 {
          tunnel: w167 -> [w176 _]
          tunnel: [w176 "Cal: Calibration failed" ("State(s) In (\"\")")] -> w164
          tunnel: w160 -> [w175 _]
          frame No Error {
            n122 = flat-sequence {
              tunnel: w175 -> [w177]
              frame #0 {
                n123 = Format Into String(format string="第%d点校准通过，按确认继续。" ("格式字符串"), w177) -> (resulting string=w179:string)  [unwired: 2 in, 1 out]
                n124 = One Button Dialog(message=w179) -> ()  [unwired: 1 in, 1 out]
              }
              frame #1 {
                n125 = Wait (ms)(milliseconds to wait=u32 2000 ("等待时间（毫秒）")) -> ()  [unwired: 1 out]
              }
            }
          }
          frame Error {
          }
        }
        n126 = call "Add State to Queue.vi"("State(s) In Front (\"\")"=w164, "State(s) In (\"\")"=w166) -> ("States Out"=w165:string)  [unwired: 13 in]
      }
      frame "Cal: Calibration failed" {
        n127 = global read "多参数全局变量.vi" "多参数编号"() -> (w261:string)
        n128 = call "Add State to Queue.vi"("State(s) In (\"\")"="init: all\nCal: Over\nidle" ("State(s) In (\"\")")) -> ("States Out"=w264:string)  [unwired: 14 in]
        n129 = Format Into String(format string="编号：%s\n参数：%s\n信息：%s" ("格式字符串"), w261, w258, "校准失败！" ("消息")) -> (resulting string=w260:string)  [unwired: 2 in, 1 out]
        n130 = One Button Dialog(message=w260) -> ()  [unwired: 1 in, 1 out]
        n131 = call "校准日志.vi"("table"="校准记录", "日志信息"=w260) -> ()  [unwired: 9 in, 1 out]
      }
      frame "Cal: Pass" {
        n132 = flat-sequence {
          tunnel: [w281] -> w271
          tunnel: w270 -> [w280]
          frame #0 {
            n133 = Wait (ms)(milliseconds to wait=u32 3000 ("等待时间（毫秒）")) -> ()  [unwired: 1 out]
          }
          frame #1 {
            n134 = case shown="1" w280 {
              tunnel: [w289 w300 w305] -> w281
              frame 0, Default {
                n135 = local read "第二点信号值"() -> (w283:dbl)
                n136 = local read "标液1"() -> (w285:sgl)
                n137 = local read "第一点校准值"() -> (w287:dbl)
                n138 = local read "第一点信号值"() -> (w288:dbl)
                n139 = local read "第二点校准值"() -> (w284:dbl)
                n140 = local read "标液2"() -> (w282:sgl)
                n141 = Format Into String(format string="校准结果：\n第一点校准值=%#.2f，第一点信号值=%#.2f，第一点标准值=%#.2f；\n第二点校准值=%#.2f，第二点信号值=%#.2f，第二点标准值=%#.2f。" ("提示"), w287, w288, w285, w284, w283, w282) -> (resulting string=w289:string)  [unwired: 2 in, 1 out]
              }
              frame 2 {
                n142 = local read "第三点信号值"() -> (w291:dbl)
                n143 = local read "第二点信号值"() -> (w294:dbl)
                n144 = local read "标液1"() -> (w296:sgl)
                n145 = local read "第三点校准值"() -> (w292:dbl)
                n146 = local read "标液3"() -> (w290:sgl)
                n147 = local read "第一点校准值"() -> (w298:dbl)
                n148 = local read "第一点信号值"() -> (w299:dbl)
                n149 = local read "第二点校准值"() -> (w295:dbl)
                n150 = local read "标液2"() -> (w293:sgl)
                n151 = Format Into String(format string="校准结果：\n第一点校准值=%#.2f，第一点信号值=%#.2f，第一点标准值=%#.2f；\n第二点校准值=%#.2f，第二点信号值=%#.2f，第二点标准值=%#.2f；\n第三点校准值=%#.2f，第三点信号值=%#.2f，第三点标准值=%#.2f。" ("提示"), w298, w299, w296, w295, w294, w293, w292, w291, w290) -> (resulting string=w300:string)  [unwired: 2 in, 1 out]
              }
              frame 1 {
                n152 = local read "第一点校准值"() -> (w304:dbl)
                n153 = local read "第一点信号值"() -> (w302:dbl)
                n154 = local read "标液1"() -> (w301:sgl)
                n155 = Format Into String(format string="校准结果：\n校准值=%#.2f，信号值=%#.2f，标准值=%#.2f。" ("提示"), w304, w302, w301) -> (resulting string=w305:string)  [unwired: 2 in, 1 out]
              }
            }
          }
        }
        n156 = call "Add State to Queue.vi"("State(s) In (\"\")"="init: all\nCal: Over\nidle" ("State(s) In (\"\")")) -> ("States Out"=w269:string)  [unwired: 14 in]
        n157 = global read "多参数全局变量.vi" "多参数编号"() -> (w275:string)
        n158 = Format Into String(format string="编号：%s\n参数：%s\n信息：%s" ("格式字符串"), w275, w274, w271) -> (resulting string=w272:string)  [unwired: 2 in, 1 out]
        n159 = One Button Dialog(message=w272) -> ()  [unwired: 1 in, 1 out]
        n160 = call "校准日志.vi"("table"="校准记录", "日志信息"=w272) -> ()  [unwired: 9 in, 1 out]
      }
      frame "Cal: Over" {
        n161 = global read "多参数全局变量.vi" "校准运行状态"() -> (w307:T7)
        n162 = Bundle By Name(cluster=w307, "叶绿素a"=FALSE ("Cond")) -> (w308:T7)
        n163 = global write "多参数全局变量.vi" "校准运行状态"(w308) -> ()
      }
      frame "idle", Default {
        n164 = event shown="[8] \"校准启动\": 值改变" {
          selector: _ -> [_ _ _ _ _ _ _ _ _ _]
          dyn-events: _ -> [_ _ _ _ _ _ _ _ _ _]
          timeout: 10 -> [_ _ _ _ _ _ _ _ _ _]
          tunnel: w320 -> [w323 w327 w332 w338 w346 w354 w359 w370 w383 _]
          tunnel: [w322 w326 w333 w342 w350 w358 w361 w372 w382 w385] -> w319
          tunnel: [w321 w324 w334 w341 w349 w357 w360 w371 w380 w386] -> w318
          tunnel: w317 -> [w321 w324 w334 w341 w349 w357 w360 w371 w380 w386]
          tunnel: [_ _ _ _ _ _ _ _ w373 _] -> _
          tunnel: w313 -> [_ _ _ w336 w344 w352 _ w366 _ _]
          event Timeout {
            n165 = event-data() -> ()  [unwired: 1 in, 3 out]
            n166 = call "Add State to Queue.vi"("State(s) In (\"\")"=w323) -> ("States Out"=w322:string)  [unwired: 14 in]
          }
          event "校准模式": Value Change {
            n167 = event-data() -> ()  [unwired: 1 in, 6 out]
            n168 = call "Add State to Queue.vi"("State(s) In (\"\")"=w327, "State(s) At Back (\"\")"="init: all\nidle" ("State(s) In (\"\")")) -> ("States Out"=w326:string)  [unwired: 13 in]
          }
          event "标液1", "标液2", "标液3", "滤波设定": Mouse Down {
            n169 = event-data() -> ("CtlRef"=w331:refnum<vi>)  [unwired: 1 in, 7 out]
            n170 = property class="DigNum (严格)"(reference=w331) -> (reference out=w328:refnum<vi>, "Value"=w329:sgl)  [unwired: 1 in, 1 out]
            n171 = call "数字键盘.vi"("OldNumber"=w329) -> ("NewNumber"=w330:dbl)  [unwired: 1 in]
            n172 = property class="DigNum (严格)"(reference=w328, "Val(Sgnl)"=w330) -> ()  [unwired: 1 in, 2 out]
            n173 = call "Add State to Queue.vi"("State(s) In (\"\")"=w332) -> ("States Out"=w333:string)  [unwired: 14 in]
          }
          event "标液1": Value Change {
            n174 = event-data() -> ("NewVal"=w339:sgl)  [unwired: 1 in, 5 out]
            n175 = global read "多参数全局变量.vi" "MB session in"() -> (w340:refnum<class "MB_Master.lvclass">)
            n176 = call "纳清叶绿素a_第一点校准数据写入.vi"("数值"=w339, "MB session in"=w340) -> ("error out"=w337:errorcluster)  [unwired: 8 in, 1 out]
            n177 = Enqueue Element At Opposite End(queue=w336, element=T1."叶绿素a" ("元素"), error in (no error)=w337) -> ()  [unwired: 1 in, 3 out]
            n178 = call "Add State to Queue.vi"("State(s) In (\"\")"=w338) -> ("States Out"=w342:string)  [unwired: 14 in]
          }
          event "标液2": Value Change {
            n179 = event-data() -> ("NewVal"=w347:sgl)  [unwired: 1 in, 5 out]
            n180 = global read "多参数全局变量.vi" "MB session in"() -> (w348:refnum<class "MB_Master.lvclass">)
            n181 = call "纳清叶绿素a_第二点校准数据写入.vi"("数值"=w347, "MB session in"=w348) -> ("error out"=w345:errorcluster)  [unwired: 8 in, 1 out]
            n182 = Enqueue Element At Opposite End(queue=w344, element=T1."叶绿素a" ("元素"), error in (no error)=w345) -> ()  [unwired: 1 in, 3 out]
            n183 = call "Add State to Queue.vi"("State(s) In (\"\")"=w346) -> ("States Out"=w350:string)  [unwired: 14 in]
          }
          event "标液3": Value Change {
            n184 = event-data() -> ("NewVal"=w355:sgl)  [unwired: 1 in, 5 out]
            n185 = global read "多参数全局变量.vi" "MB session in"() -> (w356:refnum<class "MB_Master.lvclass">)
            n186 = call "纳清叶绿素a_第三点校准数据写入.vi"("数值"=w355, "MB session in"=w356) -> ("error out"=w353:errorcluster)  [unwired: 8 in, 1 out]
            n187 = Enqueue Element At Opposite End(queue=w352, element=T1."叶绿素a" ("元素"), error in (no error)=w353) -> ()  [unwired: 1 in, 3 out]
            n188 = call "Add State to Queue.vi"("State(s) In (\"\")"=w354) -> ("States Out"=w358:string)  [unwired: 14 in]
          }
          event "滤波设定": Value Change {
            n189 = event-data() -> ()  [unwired: 1 in, 6 out]
            n190 = flat-sequence {
              frame #0 {
                n191 = global read "断电保存变量.vi" "滤波设置"() -> (w364:T4)
                n192 = local read "滤波设定"() -> (w362:sgl)
                n193 = Bundle By Name(cluster=w364, "叶绿素a"=w362) -> (w363:T4)
                n194 = global write "断电保存变量.vi" "滤波设置"(w363) -> ()
              }
              frame #1 {
                n195 = call "配置文件保存.vi"() -> ()  [unwired: 12 in]
              }
            }
            n196 = call "Add State to Queue.vi"("State(s) In (\"\")"=w359) -> ("States Out"=w361:string)  [unwired: 14 in]
          }
          event "量程": Value Change {
            n197 = event-data() -> ("NewVal"=w368:u16)  [unwired: 1 in, 5 out]
            n198 = global read "多参数全局变量.vi" "MB session in"() -> (w369:refnum<class "MB_Master.lvclass">)
            n199 = call "纳清叶绿素a_量程写入.vi"("数值"=w368, "MB session in"=w369) -> ("error out"=w367:errorcluster)  [unwired: 8 in, 1 out]
            n200 = Enqueue Element At Opposite End(queue=w366, element=T1."叶绿素a" ("元素"), error in (no error)=w367) -> ()  [unwired: 1 in, 3 out]
            n201 = call "Add State to Queue.vi"("State(s) In (\"\")"=w370) -> ("States Out"=w372:string)  [unwired: 14 in]
          }
          event "校准启动": Value Change {
            n202 = event-data() -> ()  [unwired: 1 in, 6 out]
            n203 = global read "纳清过程全局变量.vi" "叶绿素a测试值"() -> (w375:T3)
            n204 = global read "多参数全局变量.vi" "MB session in"() -> (w376:refnum<class "MB_Master.lvclass">)
            n205 = Unbundle By Name(w375) -> ("量程"=w374:u16)
            n206 = global read "多参数全局变量.vi" "校准运行状态"() -> (w378:T7)
            n207 = Bundle By Name(cluster=w378, "叶绿素a"=TRUE ("Cond")) -> (w379:T7)
            n208 = call "纳清叶绿素a_校准量程写入.vi"("数值"=w374, "MB session in"=w376) -> ("error out"=w373:errorcluster)  [unwired: 8 in, 1 out]
            n209 = global write "多参数全局变量.vi" "校准运行状态"(w379) -> ()
            n210 = call "Add State to Queue.vi"("State(s) In (\"\")"=w383, "State(s) At Back (\"\")"="init: all\nCal: Place standard solution\n Cal: Calibration process\nidle" ("State(s) In (\"\")")) -> ("States Out"=w382:string)  [unwired: 13 in]
          }
          event "校准停止": Value Change {
            n211 = event-data() -> ()  [unwired: 1 in, 6 out]
            n212 = call "Add State to Queue.vi"("State(s) In (\"\")"="init: all\nCal: Over\nidle" ("State(s) In (\"\")")) -> ("States Out"=w385:string)  [unwired: 14 in]
          }
        }
      }
    }
  }
